vi "Editor UI.vi"(8 "error in (no error)":errorcluster, 10 "Close Event":refnum<user-event>, 11 "Device in":refnum<class "Device.lvclass">) -> (0 "error out":errorcluster, 3 "Device out":refnum<class "Device.lvclass">)   [LabVIEW 2020, in "HAL.lvlib" / "Device.lvclass"]
uses:
  Device.lvclass
panel:
  # "No\nExtra\nConfig"
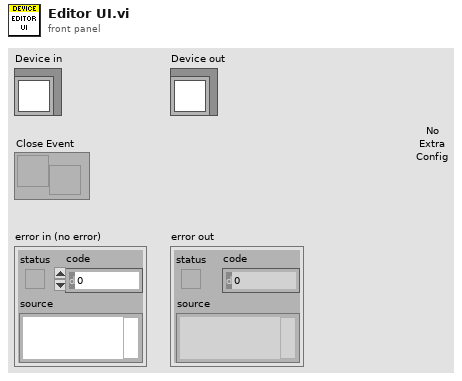
[diagram p1: front panel]
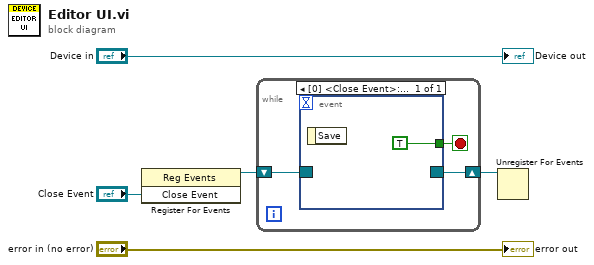
[diagram p0: block diagram]
diagram:
  n1 = register-events("Close Event") -> (reference out=w3:refnum<event-registration>)  [unwired: 2 in, 1 out]
  n2 = while {
    shift-right: [w7] -> w2
    shift-left: w3 -> [w8]
    stop <- w6 stop-if-true
    n3 = event shown="[0] <Close Event>: User Event" {
      selector: w8 -> [_]
      dyn-events: [_] -> w7
      timeout: _ -> [_]
      tunnel: [TRUE] -> w6
      event User Event {
        n4 = event-data() -> ()  [unwired: 1 in, 1 out]
      }
    }
  }
  n5 = Unregister For Events(event registration refnum=w2) -> ()  [unwired: 1 in, 1 out]
  "error out" <- "error in (no error)"
  "Device out" <- "Device in"
